vi "RtdeWriteInputs.vi"(8 "Data":T1, 10 "Rtde":refnum<k24>, 11 "error in":errorcluster) -> (3 "error out":errorcluster)   [LabVIEW 2017, in "UnderAutomation.UniversalRobots.lvlib"]
uses:
  UnderAutomation.UniversalRobots.lvlib
  C:/Users/fg/Documents/UniversalRobots.vi/LabVIEW_2024/UnderAutomation.UniversalRobots/lib/UnderAutomation.UniversalRobots.dll
  LabVIEW_2024/UnderAutomation.UniversalRobots/lib/UnderAutomation.UniversalRobots.dll
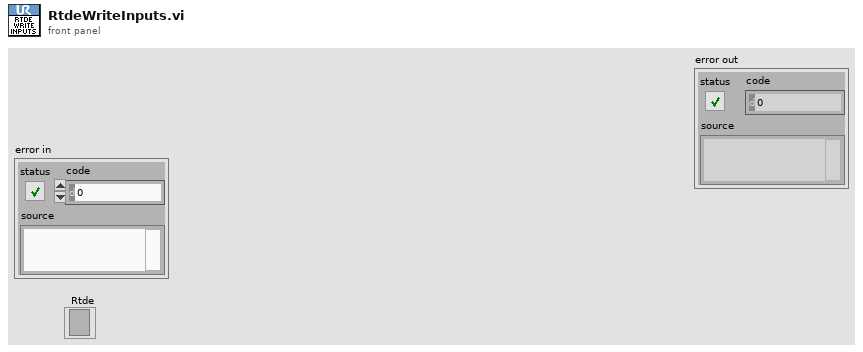
[diagram p1: front panel]
types:
  T1 = cluster{"ConfigurableDigitalOutput":u8, "ConfigurableDigitalOutputMask":u8, "ExternalForceTorque":cluster{"X":dbl, "Y":dbl, "Z":dbl, "Rx":dbl, "Ry":dbl, "Rz":dbl}, "InputBitRegisters":cluster{"X64":bool, "X65":bool, "X66":bool, "X67":bool, "X68":bool, "X69":bool, "X70":bool, "X71":bool, "X72":bool, "X73":bool, "X74":bool, "X75":bool, "X76":bool, "X77":bool, "X78":bool, "X79":bool, "X80":bool, "X81":bool, "X82":bool, "X83":bool, "X84":bool, "X85":bool, "X86":bool, "X87":bool, "X88":bool, "X89":bool, "X90":bool, "X91":bool, "X92":bool, "X93":bool, "X94":bool, "X95":bool, "X96":bool, "X97":bool, "X98":bool, "X99":bool, "X100":bool, "X101":bool, "X102":bool, "X103":bool, "X104":bool, "X105":bool, "X106":bool, "X107":bool, "X108":bool, "X109":bool, "X110":bool, "X111":bool, "X112":bool, "X113":bool, "X114":bool, "X115":bool, "X116":bool, "X117":bool, "X118":bool, "X119":bool, "X120":bool, "X121":bool, "X122":bool, "X123":bool, "X124":bool, "X125":bool, "X126":bool, "X127":bool}, "InputBtRegisters0To31":u32, "InputBtRegisters32To63":u32, "InputDoubleRegisters":cluster{"X0":dbl, "X1":dbl, "X2":dbl, "X3":dbl, "X4":dbl, "X5":dbl, "X6":dbl, "X7":dbl, "X8":dbl, "X9":dbl, "X10":dbl, "X11":dbl, "X12":dbl, "X13":dbl, "X14":dbl, "X15":dbl, "X16":dbl, "X17":dbl, "X18":dbl, "X19":dbl, "X20":dbl, "X21":dbl, "X22":dbl, "X23":dbl, "X24":dbl, "X25":dbl, "X26":dbl, "X27":dbl, "X28":dbl, "X29":dbl, "X30":dbl, "X31":dbl, "X32":dbl, "X33":dbl, "X34":dbl, "X35":dbl, "X36":dbl, "X37":dbl, "X38":dbl, "X39":dbl, "X40":dbl, "X41":dbl, "X42":dbl, "X43":dbl, "X44":dbl, "X45":dbl, "X46":dbl, "X47":dbl}, "InputIntRegisters":cluster{"X0":i32, "X1":i32, "X2":i32, "X3":i32, "X4":i32, "X5":i32, "X6":i32, "X7":i32, "X8":i32, "X9":i32, "X10":i32, "X11":i32, "X12":i32, "X13":i32, "X14":i32, "X15":i32, "X16":i32, "X17":i32, "X18":i32, "X19":i32, "X20":i32, "X21":i32, "X22":i32, "X23":i32, "X24":i32, "X25":i32, "X26":i32, "X27":i32, "X28":i32, "X29":i32, "X30":i32, "X31":i32, "X32":i32, "X33":i32, "X34":i32, "X35":i32, "X36":i32, "X37":i32, "X38":i32, "X39":i32, "X40":i32, "X41":i32, "X42":i32, "X43":i32, "X44":i32, "X45":i32, "X46":i32, "X47":i32}, "SpeedSliderFraction":dbl, "SpeedSliderMask":u32, "StandardAnalogOutput0":dbl, "StandardAnalogOutput1":dbl, "StandardAnalogOutputMask":u8, "StandardAnalogOutputType":u8, "StandardDigitalOutput":u8, "StandardDigitalOutputMask":u8}
  T2 = cluster{"X":dbl, "Y":dbl, "Z":dbl, "Rx":dbl, "Ry":dbl, "Rz":dbl}
  T3 = cluster{"X64":bool, "X65":bool, "X66":bool, "X67":bool, "X68":bool, "X69":bool, "X70":bool, "X71":bool, "X72":bool, "X73":bool, "X74":bool, "X75":bool, "X76":bool, "X77":bool, "X78":bool, "X79":bool, "X80":bool, "X81":bool, "X82":bool, "X83":bool, "X84":bool, "X85":bool, "X86":bool, "X87":bool, "X88":bool, "X89":bool, "X90":bool, "X91":bool, "X92":bool, "X93":bool, "X94":bool, "X95":bool, "X96":bool, "X97":bool, "X98":bool, "X99":bool, "X100":bool, "X101":bool, "X102":bool, "X103":bool, "X104":bool, "X105":bool, "X106":bool, "X107":bool, "X108":bool, "X109":bool, "X110":bool, "X111":bool, "X112":bool, "X113":bool, "X114":bool, "X115":bool, "X116":bool, "X117":bool, "X118":bool, "X119":bool, "X120":bool, "X121":bool, "X122":bool, "X123":bool, "X124":bool, "X125":bool, "X126":bool, "X127":bool}
  T4 = cluster{"X0":dbl, "X1":dbl, "X2":dbl, "X3":dbl, "X4":dbl, "X5":dbl, "X6":dbl, "X7":dbl, "X8":dbl, "X9":dbl, "X10":dbl, "X11":dbl, "X12":dbl, "X13":dbl, "X14":dbl, "X15":dbl, "X16":dbl, "X17":dbl, "X18":dbl, "X19":dbl, "X20":dbl, "X21":dbl, "X22":dbl, "X23":dbl, "X24":dbl, "X25":dbl, "X26":dbl, "X27":dbl, "X28":dbl, "X29":dbl, "X30":dbl, "X31":dbl, "X32":dbl, "X33":dbl, "X34":dbl, "X35":dbl, "X36":dbl, "X37":dbl, "X38":dbl, "X39":dbl, "X40":dbl, "X41":dbl, "X42":dbl, "X43":dbl, "X44":dbl, "X45":dbl, "X46":dbl, "X47":dbl}
  T5 = cluster{"X0":i32, "X1":i32, "X2":i32, "X3":i32, "X4":i32, "X5":i32, "X6":i32, "X7":i32, "X8":i32, "X9":i32, "X10":i32, "X11":i32, "X12":i32, "X13":i32, "X14":i32, "X15":i32, "X16":i32, "X17":i32, "X18":i32, "X19":i32, "X20":i32, "X21":i32, "X22":i32, "X23":i32, "X24":i32, "X25":i32, "X26":i32, "X27":i32, "X28":i32, "X29":i32, "X30":i32, "X31":i32, "X32":i32, "X33":i32, "X34":i32, "X35":i32, "X36":i32, "X37":i32, "X38":i32, "X39":i32, "X40":i32, "X41":i32, "X42":i32, "X43":i32, "X44":i32, "X45":i32, "X46":i32, "X47":i32}
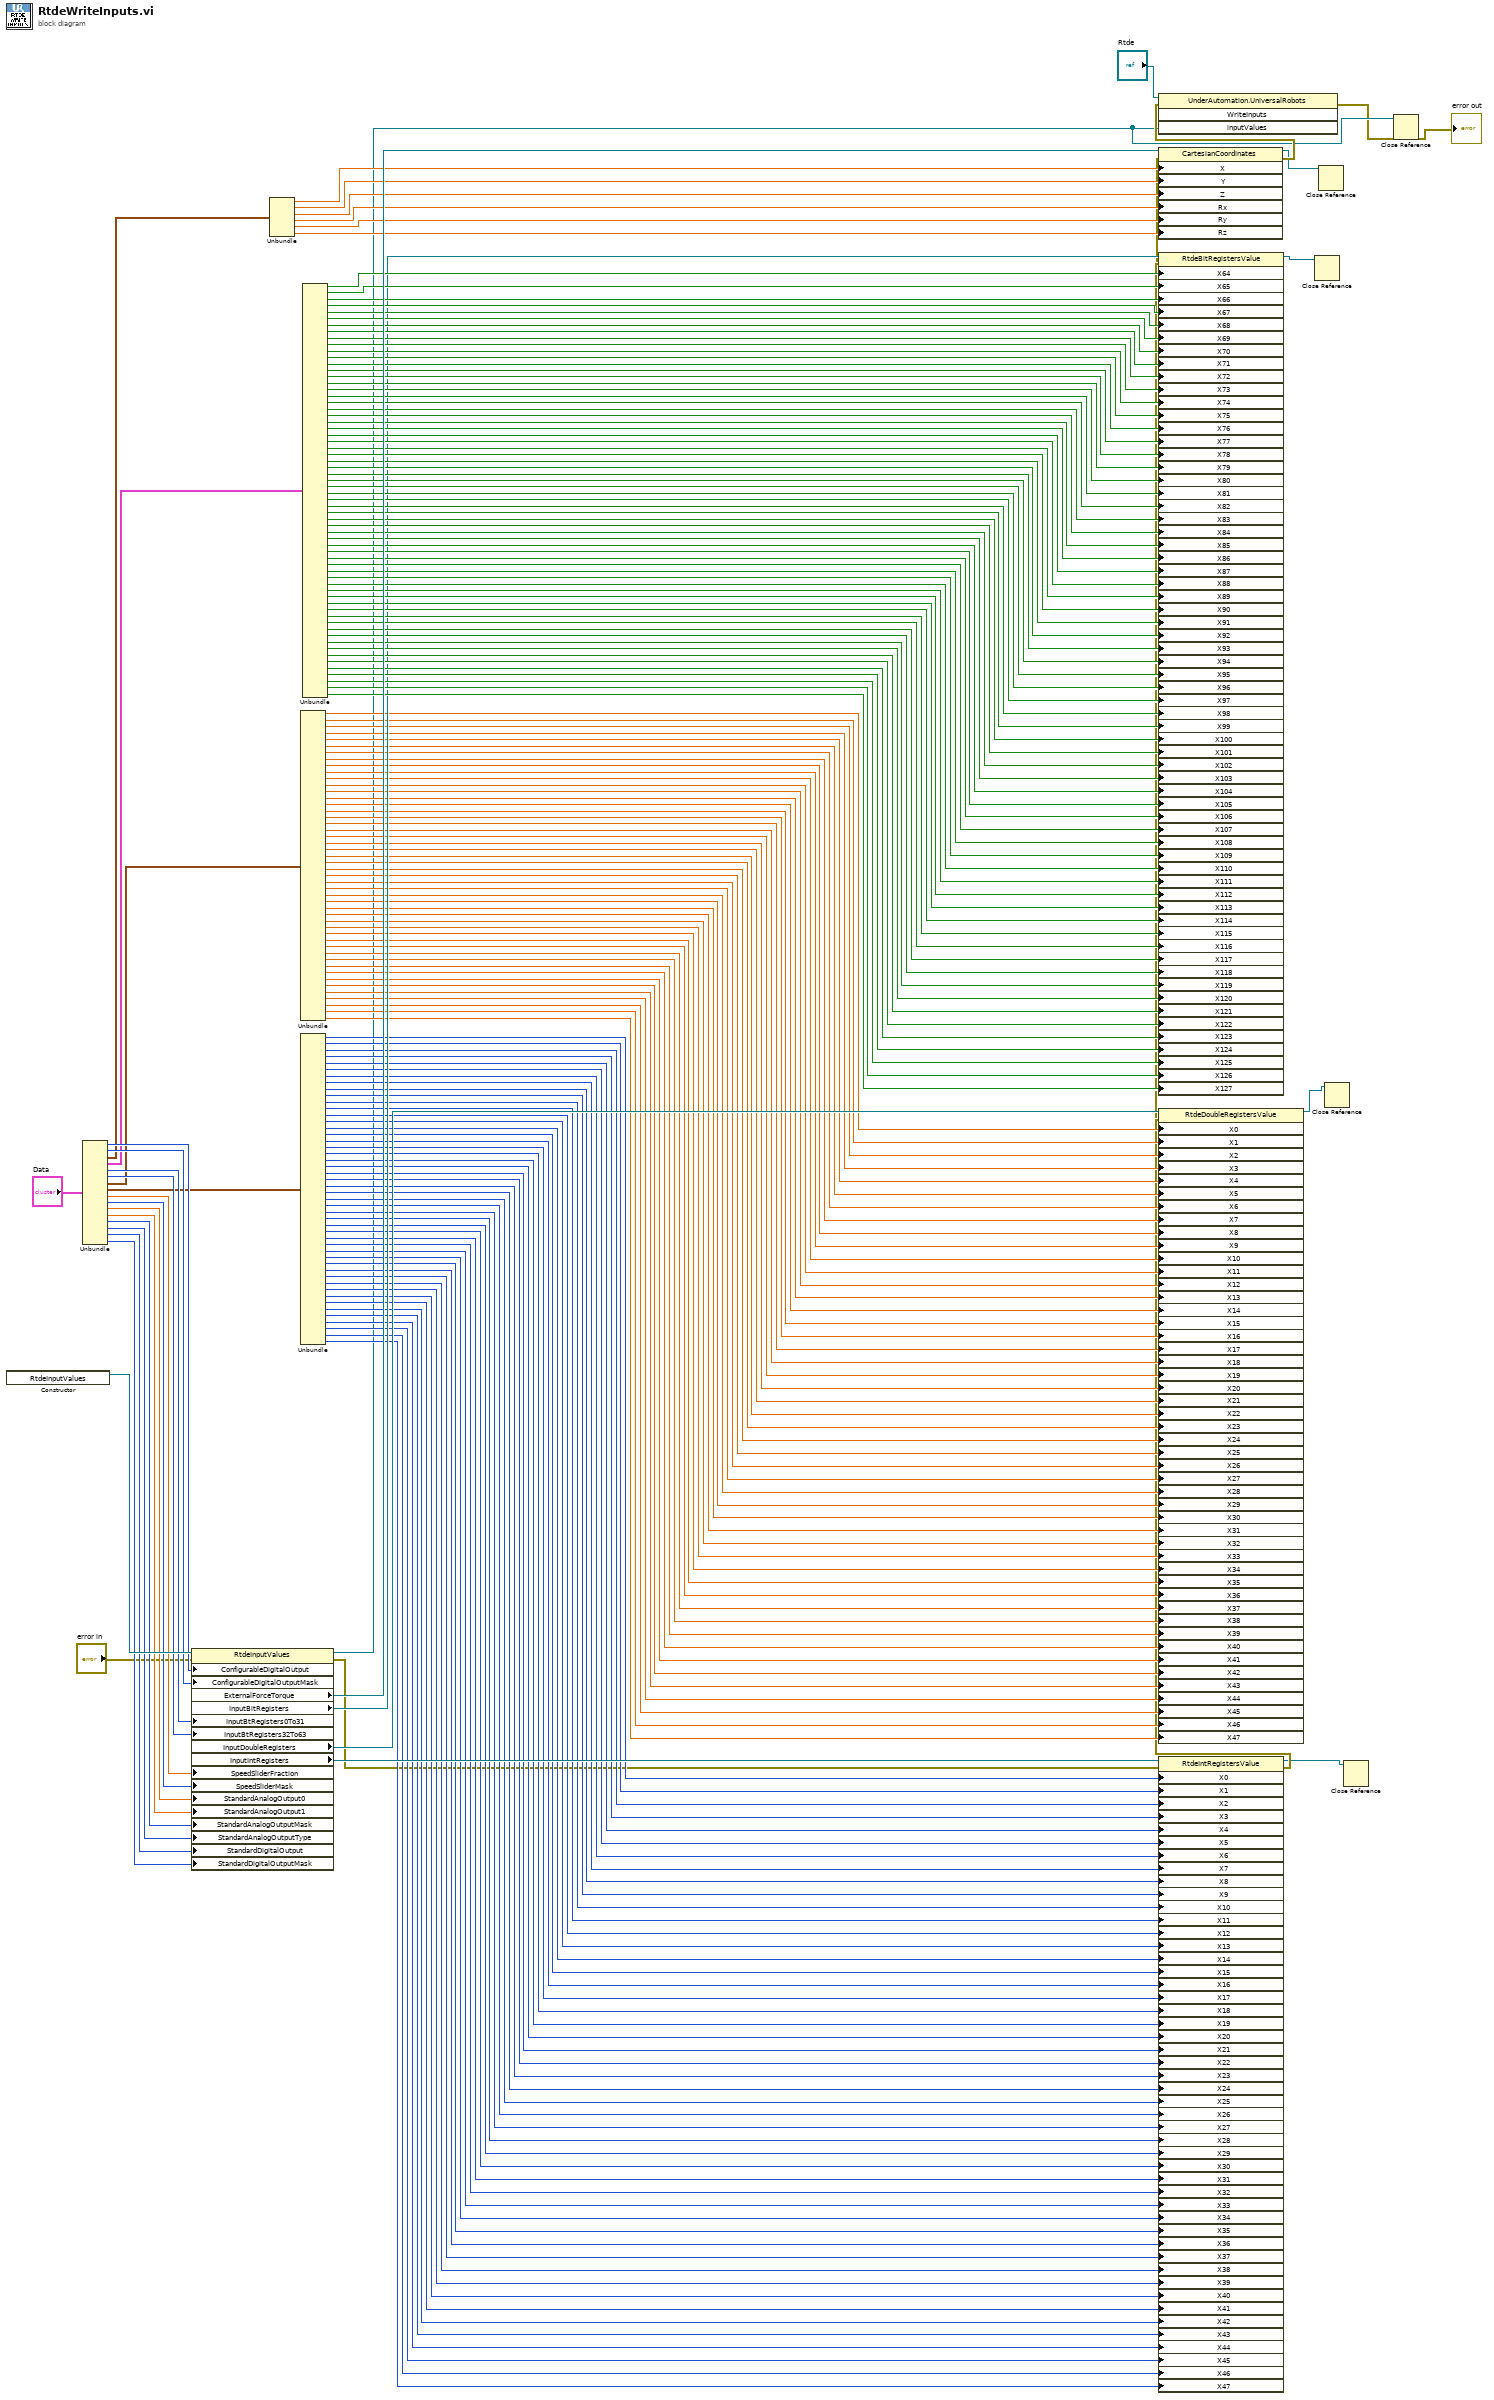
[diagram p0: block diagram]
diagram:
  n1 = constructor class="RtdeInputValues"() -> (reference out=w201:refnum<k24>)  [unwired: 3 in, 2 out]
  n2 = Unbundle("Data") -> ("ConfigurableDigitalOutput"=w199:u8, "ConfigurableDigitalOutputMask"=w198:u8, "ExternalForceTorque"=w187:T2, "InputBitRegisters"=w179:T3, "InputBtRegisters0To31"=w197:u32, "InputBtRegisters32To63"=w196:u32, "InputDoubleRegisters"=w114:T4, "InputIntRegisters"=w62:T5, "SpeedSliderFraction"=w195:dbl, "SpeedSliderMask"=w194:u32, "StandardAnalogOutput0"=w193:dbl, "StandardAnalogOutput1"=w192:dbl, "StandardAnalogOutputMask"=w191:u8, "StandardAnalogOutputType"=w190:u8, "StandardDigitalOutput"=w189:u8, "StandardDigitalOutputMask"=w188:u8)
  n3 = property class="RtdeInputValues"(reference=w201, error in="error in", "ConfigurableDigitalOutput"=w199, "ConfigurableDigitalOutputMask"=w198, "InputBtRegisters0To31"=w197, "InputBtRegisters32To63"=w196, "SpeedSliderFraction"=w195, "SpeedSliderMask"=w194, "StandardAnalogOutput0"=w193, "StandardAnalogOutput1"=w192, "StandardAnalogOutputMask"=w191, "StandardAnalogOutputType"=w190, "StandardDigitalOutput"=w189, "StandardDigitalOutputMask"=w188) -> (reference out=w7:refnum<k24>, error out=w12:errorcluster, "ExternalForceTorque"=w186:refnum<k24>, "InputBitRegisters"=w113:refnum<k24>, "InputDoubleRegisters"=w112:refnum<k24>, "InputIntRegisters"=w63:refnum<k24>)
  n4 = Unbundle(w187) -> ("X"=w185:dbl, "Y"=w184:dbl, "Z"=w182:dbl, "Rx"=w183:dbl, "Ry"=w181:dbl, "Rz"=w180:dbl)
  n5 = Unbundle(w114) -> ("X0"=w111:dbl, "X1"=w110:dbl, "X2"=w109:dbl, "X3"=w108:dbl, "X4"=w107:dbl, "X5"=w106:dbl, "X6"=w105:dbl, "X7"=w104:dbl, "X8"=w103:dbl, "X9"=w102:dbl, "X10"=w101:dbl, "X11"=w100:dbl, "X12"=w99:dbl, "X13"=w98:dbl, "X14"=w95:dbl, "X15"=w97:dbl, "X16"=w96:dbl, "X17"=w94:dbl, "X18"=w93:dbl, "X19"=w92:dbl, "X20"=w91:dbl, "X21"=w90:dbl, "X22"=w89:dbl, "X23"=w88:dbl, "X24"=w87:dbl, "X25"=w86:dbl, "X26"=w85:dbl, "X27"=w84:dbl, "X28"=w83:dbl, "X29"=w82:dbl, "X30"=w81:dbl, "X31"=w80:dbl, "X32"=w79:dbl, "X33"=w78:dbl, "X34"=w77:dbl, "X35"=w75:dbl, "X36"=w76:dbl, "X37"=w74:dbl, "X38"=w73:dbl, "X39"=w72:dbl, "X40"=w71:dbl, "X41"=w70:dbl, "X42"=w69:dbl, "X43"=w68:dbl, "X44"=w67:dbl, "X45"=w66:dbl, "X46"=w65:dbl, "X47"=w64:dbl)
  n6 = Unbundle(w62) -> ("X0"=w61:i32, "X1"=w60:i32, "X2"=w59:i32, "X3"=w58:i32, "X4"=w57:i32, "X5"=w56:i32, "X6"=w55:i32, "X7"=w54:i32, "X8"=w53:i32, "X9"=w52:i32, "X10"=w51:i32, "X11"=w50:i32, "X12"=w49:i32, "X13"=w48:i32, "X14"=w47:i32, "X15"=w46:i32, "X16"=w45:i32, "X17"=w44:i32, "X18"=w43:i32, "X19"=w42:i32, "X20"=w41:i32, "X21"=w40:i32, "X22"=w39:i32, "X23"=w38:i32, "X24"=w37:i32, "X25"=w36:i32, "X26"=w35:i32, "X27"=w34:i32, "X28"=w33:i32, "X29"=w32:i32, "X30"=w31:i32, "X31"=w30:i32, "X32"=w29:i32, "X33"=w28:i32, "X34"=w27:i32, "X35"=w26:i32, "X36"=w25:i32, "X37"=w24:i32, "X38"=w22:i32, "X39"=w23:i32, "X40"=w21:i32, "X41"=w20:i32, "X42"=w19:i32, "X43"=w18:i32, "X44"=w17:i32, "X45"=w16:i32, "X46"=w15:i32, "X47"=w14:i32)
  n7 = Unbundle(w179) -> ("X64"=w178:bool, "X65"=w177:bool, "X66"=w176:bool, "X67"=w175:bool, "X68"=w174:bool, "X69"=w173:bool, "X70"=w172:bool, "X71"=w171:bool, "X72"=w170:bool, "X73"=w169:bool, "X74"=w168:bool, "X75"=w167:bool, "X76"=w166:bool, "X77"=w165:bool, "X78"=w164:bool, "X79"=w163:bool, "X80"=w162:bool, "X81"=w161:bool, "X82"=w160:bool, "X83"=w159:bool, "X84"=w158:bool, "X85"=w157:bool, "X86"=w156:bool, "X87"=w155:bool, "X88"=w154:bool, "X89"=w153:bool, "X90"=w152:bool, "X91"=w151:bool, "X92"=w150:bool, "X93"=w149:bool, "X94"=w148:bool, "X95"=w147:bool, "X96"=w146:bool, "X97"=w145:bool, "X98"=w144:bool, "X99"=w143:bool, "X100"=w142:bool, "X101"=w141:bool, "X102"=w140:bool, "X103"=w139:bool, "X104"=w138:bool, "X105"=w137:bool, "X106"=w136:bool, "X107"=w135:bool, "X108"=w134:bool, "X109"=w133:bool, "X110"=w132:bool, "X111"=w131:bool, "X112"=w130:bool, "X113"=w129:bool, "X114"=w128:bool, "X115"=w127:bool, "X116"=w126:bool, "X117"=w125:bool, "X118"=w123:bool, "X119"=w124:bool, "X120"=w122:bool, "X121"=w121:bool, "X122"=w120:bool, "X123"=w119:bool, "X124"=w118:bool, "X125"=w117:bool, "X126"=w116:bool, "X127"=w115:bool)
  n8 = property class="RtdeIntRegistersValue"(reference=w63, error in=w12, "X0"=w61, "X1"=w60, "X2"=w59, "X3"=w58, "X4"=w57, "X5"=w56, "X6"=w55, "X7"=w54, "X8"=w53, "X9"=w52, "X10"=w51, "X11"=w50, "X12"=w49, "X13"=w48, "X14"=w47, "X15"=w46, "X16"=w45, "X17"=w44, "X18"=w43, "X19"=w42, "X20"=w41, "X21"=w40, "X22"=w39, "X23"=w38, "X24"=w37, "X25"=w36, "X26"=w35, "X27"=w34, "X28"=w33, "X29"=w32, "X30"=w31, "X31"=w30, "X32"=w29, "X33"=w28, "X34"=w27, "X35"=w26, "X36"=w25, "X37"=w24, "X38"=w22, "X39"=w23, "X40"=w21, "X41"=w20, "X42"=w19, "X43"=w18, "X44"=w17, "X45"=w16, "X46"=w15, "X47"=w14) -> (reference out=w1:refnum<k24>, error out=w11:errorcluster)
  n9 = property class="RtdeDoubleRegistersValue"(reference=w112, error in=w11, "X0"=w111, "X1"=w110, "X2"=w109, "X3"=w108, "X4"=w107, "X5"=w106, "X6"=w105, "X7"=w104, "X8"=w103, "X9"=w102, "X10"=w101, "X11"=w100, "X12"=w99, "X13"=w98, "X14"=w95, "X15"=w97, "X16"=w96, "X17"=w94, "X18"=w93, "X19"=w92, "X20"=w91, "X21"=w90, "X22"=w89, "X23"=w88, "X24"=w87, "X25"=w86, "X26"=w85, "X27"=w84, "X28"=w83, "X29"=w82, "X30"=w81, "X31"=w80, "X32"=w79, "X33"=w78, "X34"=w77, "X35"=w75, "X36"=w76, "X37"=w74, "X38"=w73, "X39"=w72, "X40"=w71, "X41"=w70, "X42"=w69, "X43"=w68, "X44"=w67, "X45"=w66, "X46"=w65, "X47"=w64) -> (reference out=w2:refnum<k24>, error out=w10:errorcluster)
  n10 = property class="RtdeBitRegistersValue"(reference=w113, error in=w10, "X64"=w178, "X65"=w177, "X66"=w176, "X67"=w175, "X68"=w174, "X69"=w173, "X70"=w172, "X71"=w171, "X72"=w170, "X73"=w169, "X74"=w168, "X75"=w167, "X76"=w166, "X77"=w165, "X78"=w164, "X79"=w163, "X80"=w162, "X81"=w161, "X82"=w160, "X83"=w159, "X84"=w158, "X85"=w157, "X86"=w156, "X87"=w155, "X88"=w154, "X89"=w153, "X90"=w152, "X91"=w151, "X92"=w150, "X93"=w149, "X94"=w148, "X95"=w147, "X96"=w146, "X97"=w145, "X98"=w144, "X99"=w143, "X100"=w142, "X101"=w141, "X102"=w140, "X103"=w139, "X104"=w138, "X105"=w137, "X106"=w136, "X107"=w135, "X108"=w134, "X109"=w133, "X110"=w132, "X111"=w131, "X112"=w130, "X113"=w129, "X114"=w128, "X115"=w127, "X116"=w126, "X117"=w125, "X118"=w123, "X119"=w124, "X120"=w122, "X121"=w121, "X122"=w120, "X123"=w119, "X124"=w118, "X125"=w117, "X126"=w116, "X127"=w115) -> (reference out=w3:refnum<k24>, error out=w9:errorcluster)
  n11 = property class="CartesianCoordinates"(reference=w186, error in=w9, "X"=w185, "Y"=w184, "Z"=w182, "Rx"=w183, "Ry"=w181, "Rz"=w180) -> (reference out=w4:refnum<k24>, error out=w8:errorcluster)
  n12 = invoke class="UnderAutomation.UniversalRobots" method="WriteInputs"(reference="Rtde", error in=w8, "inputValues"=w7) -> (error out=w6:errorcluster)  [unwired: 1 in, 3 out]
  n13 = Close Reference(reference=w3) -> ()  [unwired: 1 in, 1 out]
  n14 = Close Reference(reference=w4) -> ()  [unwired: 1 in, 1 out]
  n15 = Close Reference(reference=w2) -> ()  [unwired: 1 in, 1 out]
  n16 = Close Reference(reference=w1) -> ()  [unwired: 1 in, 1 out]
  n17 = Close Reference(reference=w7, error in (no error)=w6) -> (error out=→"error out":errorcluster)
